vi "DoWrite.vi"(7 "LabVIEW Web Service Request":refnum<class "Web Request.lvclass">) -> ()   [LabVIEW 2018]
uses:
  <vilib>/wsapi/Web Request.lvclass
  CAEN globals.vi
panel:
  in  "error in (no error)":errorcluster
  # "Use the Web Service Request input terminal to call the VIs on the Web Services palette. Do not remove it from the connector pane unless you don't need access to the palette."
  # "Each additional control wired to the connector pane will be available as an input in the URL. To include an indicator in terminal-mode output (the default setting), it must also be wired to the connector pane."
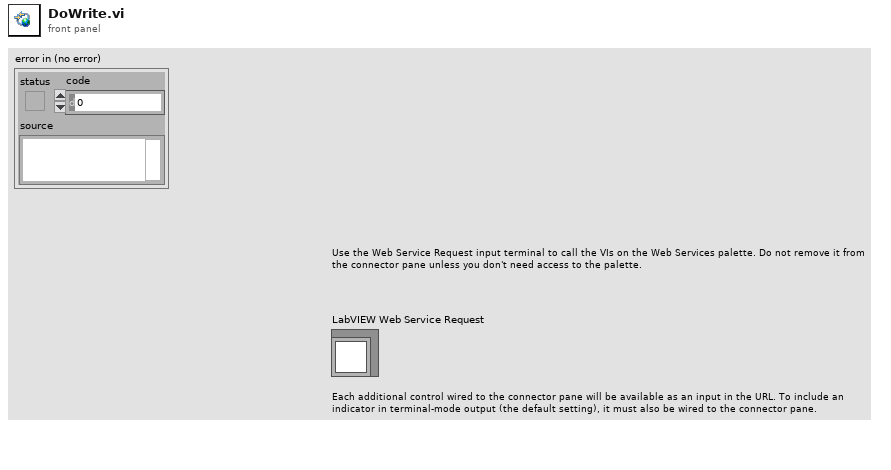
[diagram p1: front panel]
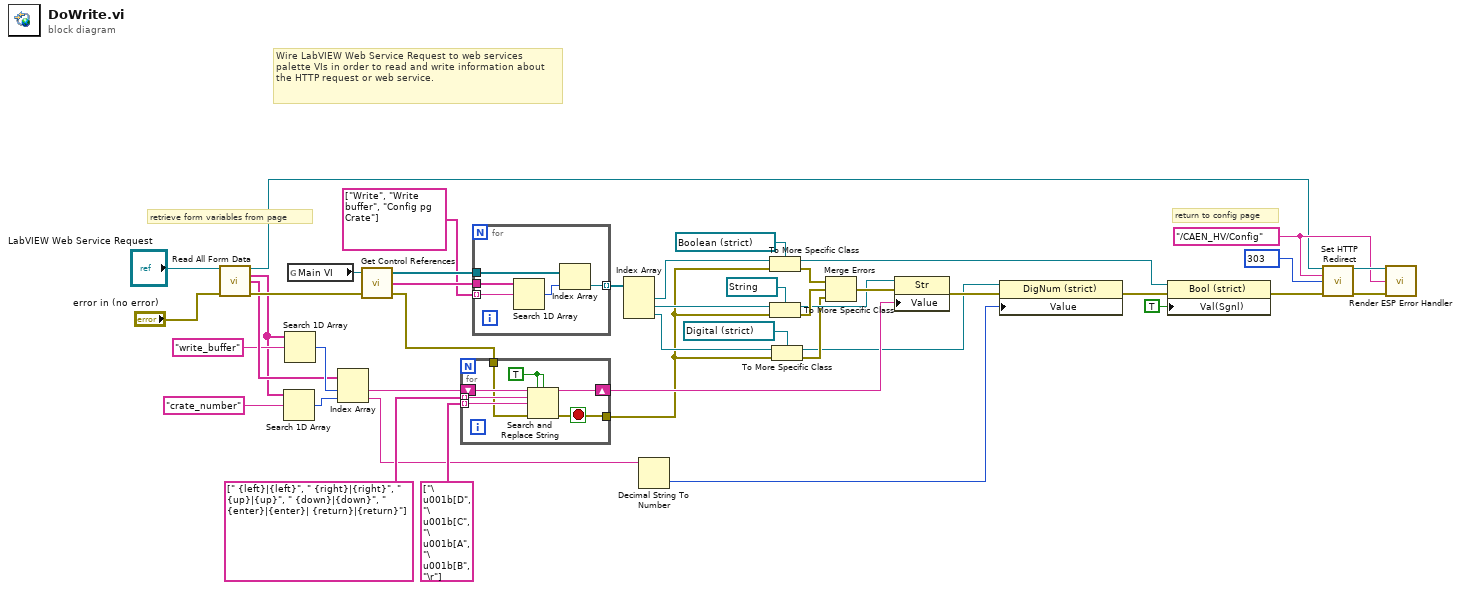
[diagram p0: block diagram]
diagram:
  w41 = 303 items=["100"=100, "101"=101, "200"=200, "201"=201, "202"=202, "203"=203, "204"=204, "205"=205, "206"=206, "300"=300, "301"=301, "302"=302, "303"=303, "304"=304, "305"=305, "306"=306, "307"=307, "400"=400, "401"=401, "402"=402, "403"=403, "404"=404, "405"=405, "406"=406, "407"=407, "408"=408, "409"=409, "410"=410, "411"=411, "412"=412, "413"=413, "414"=414, "415"=415, "416"=416, "417"=417, "500"=500, "501"=501, "502"=502, "503"=503, "504"=504, "505"=505] ("response code (307)")
  w38 = "/CAEN_HV/Config" ("redirect URL")
  # "retrieve form variables from page"
  # "return to config page"
  # "Wire LabVIEW Web Service Request to web services palette VIs in order to read and write information about the HTTP request or web service."
  n1 = call <vilib>:"Read All Form Data.vi"("LabVIEW Web Service Request"="LabVIEW Web Service Request", "error in (no error)"="error in (no error)") -> ("LabVIEW Web Service Request out"=w34:refnum<class "Web Request.lvclass">, "Key"=w2:string[], "Value"=w32:string[], "error out"=w35:errorcluster)  [unwired: 9 in, 1 out]
  n2 = Search 1D Array(1D array=w2, element="crate_number") -> (index of element=w4:i32)  [unwired: 1 in]
  n3 = Search 1D Array(1D array=w2, element="write_buffer") -> (index of element=w33:i32)  [unwired: 1 in]
  n4 = global read "CAEN globals.vi" "Main VI"() -> (w44:refnum<vi>)
  n5 = Index Array(array=w32, index #1=w33, index #2=w4) -> (element #1=w15:string, element #2=w3:string)
  n6 = call "Get Control References.vi"("error in"=w35, "This vi"=w44) -> ("error out"=w14:errorcluster, "Control Names"=w43:string[], "Controls[]"=w42:refnum<vi>[])  [unwired: 1 in]
  n7 = for {
    tunnel: string[] [" {left}|{left}", " {right}|{right}", " {up}|{up}", " {down}|{down}", " {enter}|{enter}| {return}|{return}"] ("Value") -> [w50] mode=indexing
    shift-right: [w48] -> w13
    shift-left: w15 -> [w51]
    tunnel: [w47] -> w8
    tunnel: string[] ["\u001b[D", "\u001b[C", "\u001b[A", "\u001b[B", "\r"] ("Value") -> [w46] mode=indexing
    tunnel: w14 -> [w45]
    stop <- w47 stop-if-true
    w49 = TRUE ("replace all? (F)")
    n8 = Search and Replace String(replace all?=w49, case sensitive?=w49, input string=w51, search string=w50, replace string=w46, error in=w45) -> (result string=w48:string, error out=w47:errorcluster)  [unwired: 2 in, 2 out]
  }
  n9 = for {
    tunnel: w43 -> [w56]
    tunnel: w42 -> [w55]
    tunnel: [w53] -> w27 mode=indexing
    tunnel: string[] ["Write", "Write buffer", "Config pg Crate"] ("Value") -> [w52] mode=indexing
    n10 = Search 1D Array(1D array=w56, element=w52) -> (index of element=w54:i32)  [unwired: 1 in]
    n11 = Index Array(array=w55, index=w54) -> (element=w53:refnum<vi>)
  }
  n12 = Index Array(array=w27) -> (element #1=w25:refnum<vi>, element #2=w26:refnum<vi>, element #3=w9:refnum<vi>)  [unwired: 3 in]
  n13 = Decimal String To Number(string=w3) -> (number=w5:i32)  [unwired: 2 in, 1 out]
  n14 = To More Specific Class(target class=refnum<vi> refnum ("replace all? (F)"), reference=w25, error in=w8) -> (specific class reference=w20:refnum<vi>, error out=w24:errorcluster)
  n15 = To More Specific Class(target class=refnum<vi> refnum ("Label.Text"), reference=w26, error in=w8) -> (specific class reference=w21:refnum<vi>, error out=w23:errorcluster)
  n16 = To More Specific Class(target class=refnum<vi> refnum ("Config pg Crate"), reference=w9, error in=w8) -> (specific class reference=w7:refnum<vi>, error out=w10:errorcluster)
  n17 = Merge Errors(w24, w23, w10) -> (w22:errorcluster)
  n18 = property class="Str"(reference=w21, error in=w22, "Value"=w13) -> (error out=w12:errorcluster)  [unwired: 1 out]
  n19 = property class="DigNum (strict)"(reference=w7, error in=w12, "Value"=w5) -> (error out=w11:errorcluster)  [unwired: 1 out]
  n20 = property class="Bool (strict)"(reference=w20, error in=w11, "Val(Sgnl)"=TRUE ("Value")) -> (error out=w19:errorcluster)  [unwired: 1 out]
  n21 = call <vilib>:"Set HTTP Redirect.vi"("LabVIEW Web Service Request"=w34, "redirect URL"=w38, "response code (307)"=w41, "error in (no error)"=w19) -> ("LabVIEW Web Service Request out"=w39:refnum<class "Web Request.lvclass">, "error out"=w40:errorcluster)  [unwired: 10 in]
  n22 = call "Render ESP Error Handler.vi"("LabVIEW Web Service Request"=w39, "Link"=w38, "error in (no error)"=w40) -> ()  [unwired: 11 in, 2 out]
